vi "cluster_v40.vi"() -> ()   [LabVIEW 2010]
panel:
  in  "Reset Signal":bool
  in  "stop":bool
  in  "Faza":dbl(slide)=107.29411764705883 scale=0.0..360.0
  in  "Frecventa":dbl(knob)=28.751924365486083 min=0.0 max=10.0 step=1.0 scale=0.0..100.0
  out "Waveform Graph":dynamicdata(graph)=[{"t0"=timestamp(8.700000000000001 s since 1904-01-01), "dt"=0.001, "Y"=[-4.864040141276061, -4.256893450931275, -3.5111972797148456, -2.6512218656773445, -1.7049569033109346, -0.7032005605317573, 0.32144291196616204, 1.3356243540900206, 2.306335114358262, 3.201981385347245, 3.9934124900854804, 4.6548696516688475, 5.16482436640972, 5.506679093916304, 5.669307458681317, 5.647416381191983, 5.441718352248652, 5.058908243464848, 4.5114454086993785, 3.8171481683841773, 2.998613875101611, 2.082483435587353, 1.0985742268249923, 0.07890962728763817, -0.9433232507425908, -1.9348537050003969, -2.86341030767361, -3.6987712463670492, -4.413747956055415, -4.985070027670572, -5.394142592126595, -5.627651529138936, -5.67799680305369, -5.543539821868113, -5.228656768626849, -4.7435961694122994, -4.1041453336760885, -3.3311165233071818, -2.4496695741365633, -1.4884930165752484, -0.47887034752329843, 0.5463381563208414, 1.5537649447400725, 2.5106212105536225, 3.385764069772174, 4.150710171747912, 4.780562749261931, 5.254821935769265, 5.558051976335801, 5.680383616494769, 5.617835317729035, 5.372442844951042, 4.952193008285376, 4.370763715665978, 3.6470787967786373, 2.804692087532624, 1.8710208213176227, 0.8764532779273312, -0.14664026642230196, -1.1649610972845341, -2.145365838133021, -3.055945170716226, -3.8670623904099695, -4.552317994616875, -5.08940890967028, -5.460854390909959, -5.654564969996828, -5.664235931888996, -5.489552514949802, -5.136200155522157, -4.615679443538078, -3.944931811819329, -3.1457881417919324, -2.2442582318923394, -1.2696842543986717, -0.2537857532011408, 0.770372734947895, 1.7694578347833596, 2.7109522367873193, 3.5642130408860915, 4.301469093580368, 4.898724858090174, 5.33654139917452, 5.600669063845035, 5.682511266059391, 5.579404280553877, 5.294703939340892, 4.837676409152993, 4.223196604709436, 3.471264053574896, 2.606351969798779, 1.656610722092005, 0.6529516213316052, -0.3719591525591123, -1.3847637396057029, -2.352498300948391, -3.243665895768458, -4.029261614956672, -4.683716606409228, -5.18573026667791], "attributes"=variant("NI_ChannelName"=variant(string "Sine"), "NI_ExpIsRelativeTime"=variant(bool TRUE), "NI_ExpStartTimeStamp"=variant(timestamp timestamp(3685589973.4396873 s since 1904-01-01)), "NI_ExpTimeStamp"=variant(timestamp timestamp(3685589982.139687 s since 1904-01-01)), "NI_ExpXDimension"=variant(string "t"))}]
  in  "Amplitudine":dbl(slide)=5.682819383259912 scale=0.0..10.0 scale format="%#1_6g"
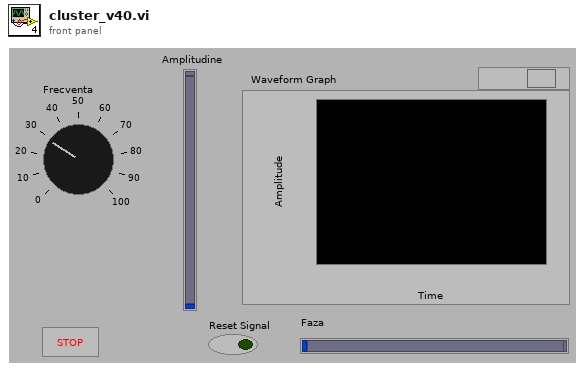
[diagram p1: front panel]
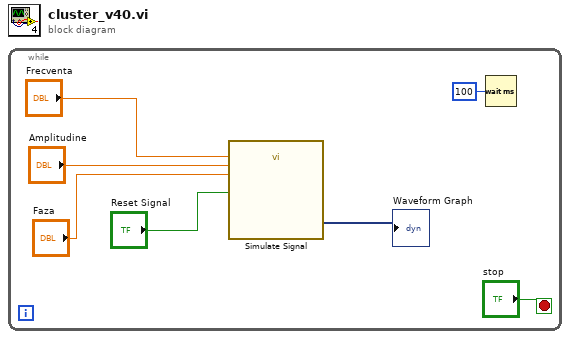
[diagram p0: block diagram]
diagram:
  n1 = while {
    stop <- "stop" stop-if-true
    n2 = call "Simulate Signal"("Reset Signal"="Reset Signal", "Frequency"="Frecventa", "Amplitude"="Amplitudine", "Phase"="Faza") -> ("Sine"=→"Waveform Graph":dynamicdata)  [unwired: 10 in, 1 out]
    n3 = Wait (ms)(milliseconds to wait=u32 100) -> ()  [unwired: 1 out]
  }
